vi "Build Signals.vi"(5 "WCM_corrections":bool, 7 "WCM_corr_coff":sgl[](array[numeric]), 8 "error in (no error)":errorcluster, 9 "II channel seq":cluster{"BG":i32[], "Ie":i32[], "I0":i32[]}[](array[cluster]), 10 "I channel seq":cluster{"BG":i32[], "Ie":i32[], "I0":i32[]}[](array[cluster]), 11 "UV-VIS in":refnum<class "UV-VIS.lvclass">) -> (0 "error out":errorcluster, 1 "Signals so Send":T1, 2 "Signals":cluster{"wavelengths":dbl[], "Tableau":dbl[]}[](array[cluster]), 3 "UV-VIS out":refnum<class "UV-VIS.lvclass">, 4 "#PP":i32)   [LabVIEW 2015]
uses:
  Detector.lvclass
  <vilib>/Analysis/NI_AALBase.lvlib
  <vilib>/Analysis/baseanly.llb/Mean (DBL).vi
  dependecies/ControlsVIs/Clusters-def/Def_signals_from_DET.ctl
  UV-VIS.lvclass
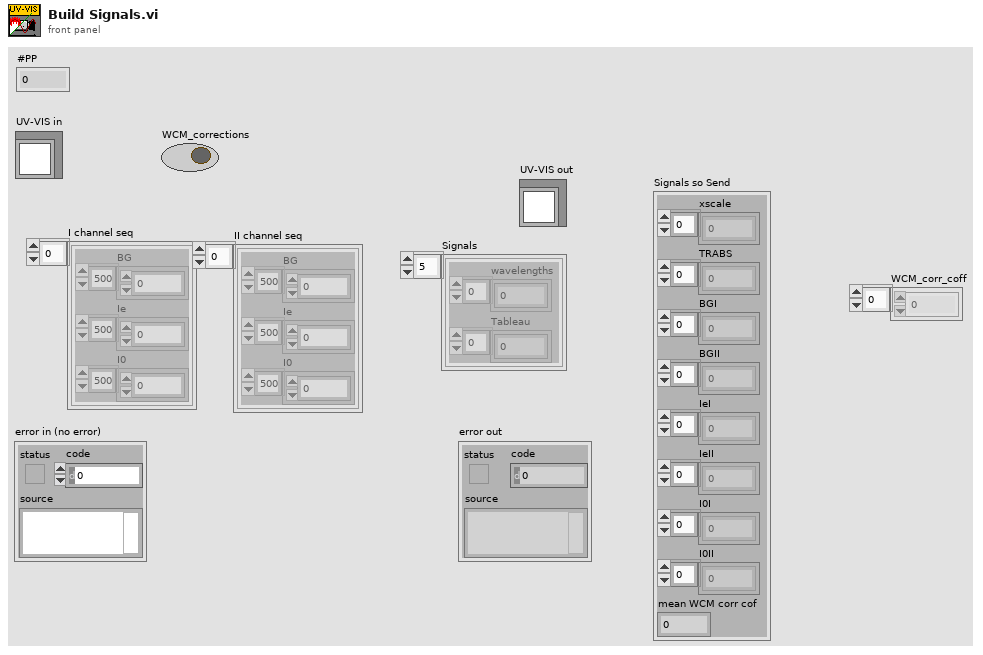
[diagram p1: front panel]
types:
  T1 = typedef "Def_signals_from_DET.ctl" = cluster{"xscale":dbl[], "TRABS":dbl[], "BGI":i32[], "BGII":i32[], "IeI":i32[], "IeII":i32[], "I0I":i32[], "I0II":i32[], "mean WCM corr cof":dbl}
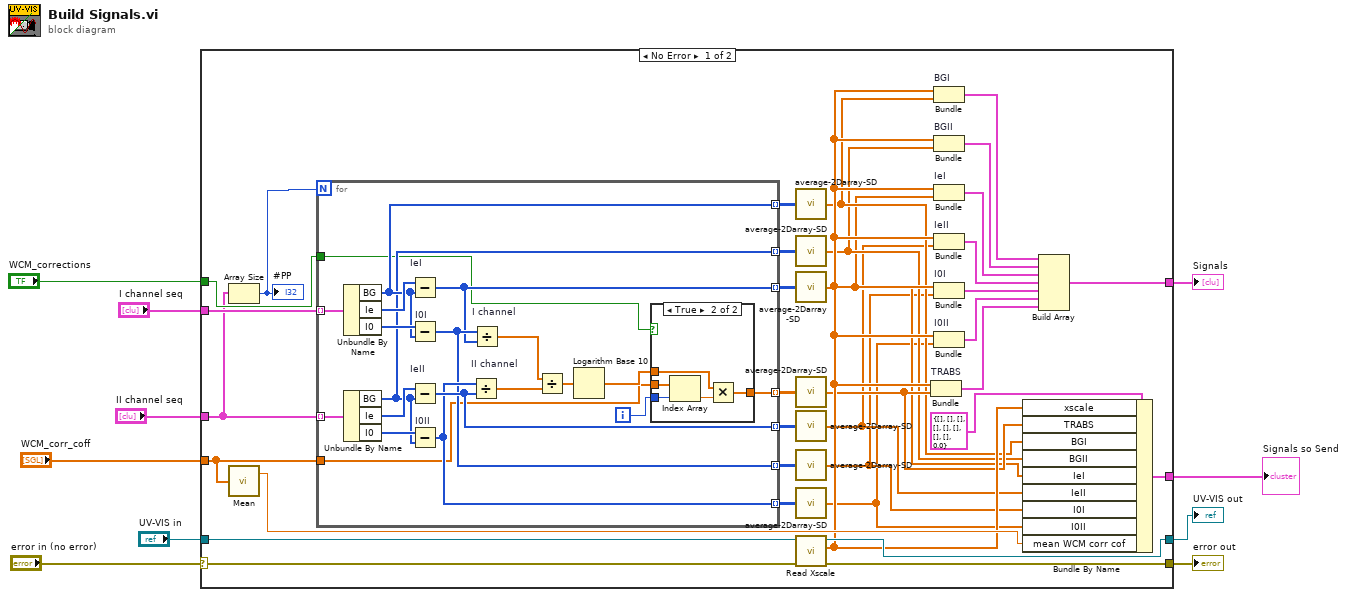
[diagram p0: block diagram]
diagram:
  n1 = case shown="No Error" "error in (no error)" {
    selector: "error in (no error)" -> [w44 w72]
    tunnel: [w39 w72] -> w9
    tunnel: [w38 w73] -> w8
    tunnel: "UV-VIS in" -> [w45 w73]
    tunnel: [w34 _] -> w6
    tunnel: "WCM_corr_coff" -> [w11 _]
    tunnel: [w32 _] -> w4
    tunnel: "I channel seq" -> [w15 _]
    tunnel: "II channel seq" -> [w13 _]
    tunnel: "WCM_corrections" -> [w14 _]
    frame No Error {
      n2 = Array Size(array=w13) -> (size(s)=w12:i32)
      "#PP" <- w12
      n3 = call-poly <vilib>:"Mean.vi"("X"=w11) -> ("mean"=w31:dbl)  [unwired: 1 out]
      n4 = for {
        N: w12 -> [_]
        tunnel: w15 -> [w65] mode=indexing
        tunnel: w13 -> [w64] mode=indexing
        tunnel: [w50] -> w22 mode=indexing
        tunnel: [w56] -> w21 mode=indexing
        tunnel: [w55] -> w20 mode=indexing
        tunnel: [w54] -> w19 mode=indexing
        tunnel: [w53] -> w18 mode=indexing
        tunnel: [w52] -> w17 mode=indexing
        tunnel: [w51] -> w16 mode=indexing
        tunnel: w14 -> [w48]
        tunnel: w11 -> [w47]
        i -> [w46]
        n5 = Unbundle By Name(w65) -> ("BG"=w53:i32[], "Ie"=w62:i32[], "I0"=w61:i32[])
        n6 = Unbundle By Name(w64) -> ("BG"=w52:i32[], "Ie"=w60:i32[], "I0"=w63:i32[])
        n7 = Subtract "IeI"(x=w62, y=w53) -> (x-y=w51:i32[])
        n8 = Subtract "I0I"(x=w61, y=w53) -> (x-y=w54:i32[])
        n9 = Subtract "IeII"(x=w60, y=w52) -> (x-y=w56:i32[])
        n10 = Subtract "I0II"(x=w63, y=w52) -> (x-y=w55:i32[])
        n11 = Divide "II channel"(x=w55, y=w56) -> (x/y=w57:dbl[])
        n12 = Divide "I channel"(x=w54, y=w51) -> (x/y=w58:dbl[])
        n13 = Divide(x=w58, y=w57) -> (x/y=w59:dbl[])
        n14 = Logarithm Base 10(1:w59) -> (0:w49:dbl[])
        n15 = case shown="True" w48 {
          tunnel: [w66 w70] -> w50
          tunnel: w49 -> [w66 w71]
          tunnel: w47 -> [_ w69]
          tunnel: w46 -> [_ w68]
          frame False {
          }
          frame True {
            n16 = Index Array(array=w69, index=w68) -> (element=w67:sgl)
            n17 = Multiply(x=w71, y=w67) -> (x*y=w70:dbl[])
          }
        }
      }
      n18 = call "average-2Darray-SD.vi"("2D array"=w18) -> ("out array"=w28:dbl[])
      n19 = call "average-2Darray-SD.vi"("2D array"=w17) -> ("out array"=w27:dbl[])
      n20 = call "average-2Darray-SD.vi"("2D array"=w16) -> ("out array"=w26:dbl[])
      n21 = call "average-2Darray-SD.vi"("2D array"=w22) -> ("out array"=w29:dbl[])
      n22 = call "average-2Darray-SD.vi"("2D array"=w21) -> ("out array"=w25:dbl[])
      n23 = call "average-2Darray-SD.vi"("2D array"=w19) -> ("out array"=w24:dbl[])
      n24 = call "average-2Darray-SD.vi"("2D array"=w20) -> ("out array"=w23:dbl[])
      n25 = call "Read Xscale.vi"("error in (no error)"=w44, "Detector en entrée"=w45) -> ("error out"=w39:errorcluster, "Xscale"=w30:dbl[], "Detector en sortie"=w38:refnum<class "UV-VIS.lvclass">)  [unwired: 7 in]
      n26 = Bundle "TRABS"("Xscale"=w30, "out array"=w29) -> (w35:cluster{"Xscale":dbl[], "out array":dbl[]})  [unwired: 1 in]
      n27 = Bundle "BGI"("Xscale"=w30, "out array"=w28) -> (w42:cluster{"Xscale":dbl[], "out array":dbl[]})  [unwired: 1 in]
      n28 = Bundle "BGII"("Xscale"=w30, "out array"=w27) -> (w43:cluster{"Xscale":dbl[], "out array":dbl[]})  [unwired: 1 in]
      n29 = Bundle "IeI"("Xscale"=w30, "out array"=w26) -> (w41:cluster{"Xscale":dbl[], "out array":dbl[]})  [unwired: 1 in]
      n30 = Bundle "IeII"("Xscale"=w30, "out array"=w25) -> (w40:cluster{"Xscale":dbl[], "out array":dbl[]})  [unwired: 1 in]
      n31 = Bundle "I0I"("Xscale"=w30, "out array"=w24) -> (w37:cluster{"Xscale":dbl[], "out array":dbl[]})  [unwired: 1 in]
      n32 = Bundle "I0II"("Xscale"=w30, "out array"=w23) -> (w36:cluster{"Xscale":dbl[], "out array":dbl[]})  [unwired: 1 in]
      n33 = Bundle By Name(cluster=T1 {"xscale"=[], "TRABS"=[], "BGI"=[], "BGII"=[], "IeI"=[], "IeII"=[], "I0I"=[], "I0II"=[], "mean WCM corr cof"=0.0}, "xscale"=w30, "TRABS"=w29, "BGI"=w28, "BGII"=w27, "IeI"=w26, "IeII"=w25, "I0I"=w24, "I0II"=w23, "mean WCM corr cof"=w31) -> (w32:T1)
      n34 = Build Array(w42, w43, w41, w40, w37, w36, w35) -> (w34:cluster{"Xscale":dbl[], "out array":dbl[]}[])
    }
    frame Error {
    }
  }
  "error out" <- w9
  "UV-VIS out" <- w8
  "Signals" <- w6
  "Signals so Send" <- w4
